vi "grabSetup.vi"(0 "HGF_ImaqDx":refnum<class "HGF_ImaqDx.lvclass">, 5 "error in (no error)":errorcluster, 6 "Region of Interest":i32[](array[numeric]), 7 "Step x":i32=-1, 8 "Channel":i32=-1, 9 "Step y":i32=-1) -> (14 "dup HGF_ImaqDx":refnum<class "HGF_ImaqDx.lvclass">, 19 "error out":errorcluster)   [LabVIEW 2009, in "HGF_IMAQ.lvlib" / "HGF_ImaqDx.lvclass"]
doc: "Starts a grab acquisition. This VI performs a continuous acquisition that provides access to the most recently acquired image.\n\nParameter are used for framegrabber, only, and can be ignored for IMAQdx and IMAQ for USB."
uses:
  HGF_ImaqDx.lvclass
  HGF_ImaqDx.lvclass/HGF_ImaqDx.ctl
  <vilib>/vision/driver/NI_Vision_Acquisition_Software.lvlib
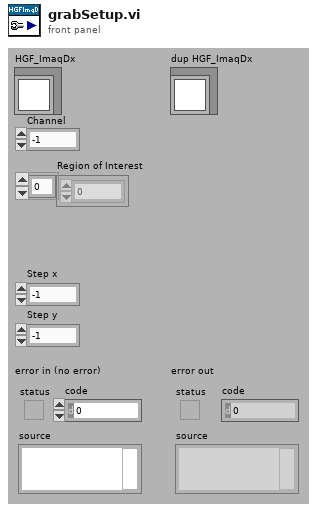
[diagram p1: front panel]
types:
  T1 = typedef "IMAQdx.ctl" = refnum<k21>
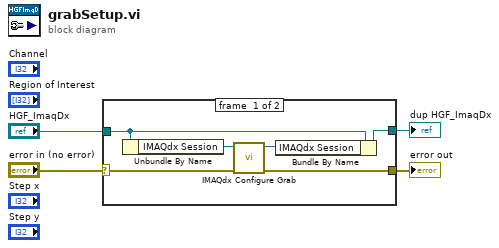
[diagram p0: block diagram]
diagram:
  n1 = case shown="No Error" "error in (no error)" {
    selector: "error in (no error)" -> [w5 w11]
    tunnel: "HGF_ImaqDx" -> [w9 w12]
    tunnel: [w7 w12] -> w3
    tunnel: [w6 w11] -> w2
    frame #0 {
      n2 = Unbundle By Name(w9) -> ("IMAQdx Session"=w10:T1)
      n3 = call <vilib>:"IMAQdx Configure Grab.vi"("error in"=w5, "Session In"=w10) -> ("error out"=w6:errorcluster, "Session Out"=w8:T1)  [unwired: 8 out]
      n4 = Bundle By Name(cluster=w9, "IMAQdx Session"=w8) -> (w7:refnum<class "HGF_ImaqDx.lvclass">)
    }
    frame #1 {
    }
  }
  "error out" <- w2
  "dup HGF_ImaqDx" <- w3
